vi "Load Program Definition as Table.vi"() -> ()   [LabVIEW 2010]
doc: "This function is an offline tool for importing MICS Command and Response Tables from Excel. \n\nInstructions\n1) Copy clipboard from Excel to Import Control.\n2) Run VI.\n3) Edit - Make Current Values Defaults.\n4) Save VI.\n5) Copy tables to new VIs."
panel:
  out "error out":errorcluster
  in  "error in":errorcluster
  in  "Table 2":string[][](table)=[["255", "0xFF", "COMMAND ACCEPTED", "The received command (identified in the response) was processed and performed without error. Any data to be returned as a result of the command completion is present in the response."], ["0", "0x00", "INVALID EXID", "The External ID contained in the command is for an external device the xPG has not been configured to process commands from."], ["1", "0x01", "INVALID COMMAND", "The Token in the received command is invalid/unknown to the xPG."], ["2", "0x02", "INVALID PARAM", "A parameter provided with the received command has been determined to be invalid and prohibits further processing of the command."], ["3", "0x03", "BUSY", "The xPG cannot execute the received command while in its present operational state.  Examples include: * Selecting program while stim on * Restoring program defaults while stim on * Writing to flash while stim on [CP commands] "], ["16", "0x10", "COMMAND NOT VALID WHILE IDLE", "The command is not valid when stimulation is not active.  (This code generally applies to commands that are used to modify stimulation.)"], ["17", "0x11", "COMMAND NOT VALID WHILE RAMPING", "The command is not valid when the xPG is ramping the stimulus amplitude immediately after turning stimulation on.  (This code generally applies to commands that are used to modify stimulation parameters)"], ["18", "0x12", "COMMAND LOCKED OUT (temporary)", "The command is temporarily locked out. (This code generally applies to commands that are used to modify stimulation, resulting in an increase in stimulation energy)"], ["19", "0x13", "DEPRECATED", ""], ["32", "0x20", "PROGRAM NOT VALID", "The command cannot be executed because the program definition is not valid.  A way to delete a program is to set it not valid.  Then when IPG returns valid programs bitmap it will not be listed as available."], ["33", "0x21", "PROGRAM DISABLED", "The command cannot be executed because the program definition has been disabled, due to a hardware issue."], ["34", "0x22", "BATTERY TOO LOW", "The xPG Stimulation command to turn stimulation on cannot be executed because the battery level is too low for safe stimulation.  IPG could have said battery was OK, but then dropped below threshold since having last sent status.  "], ["35", "0x23", "DEPRECATED –  Use 0x03 BUSY. ", ""], ["36", "0x24", "NO PROGRAM SELECTED", "The requested command (only in response to stim on) cannot be executed because no program is presently selected."], ["37", "0x25", "BOOST CONVERTER STARTUP FAILED", "Stimulation cannot be started because the high voltage boost converter did not initialize correctly."], ["38", "0x26", "PULSE GUARD CHECK FAILED", "Stimulation cannot be started because the pulse guard circuit check failed."], ["39", "0x27", "STIMULATION POWER ON FAILED", "Stimulation cannot be started because the stimulation chip failed to power up correctly."], ["40", "0x28", "ACTIVE RECOVERY DISABLED", "Stimulation cannot be started because automatic waveform adjustment failed."], ["41", "0x29", "DEPRECATED – Use 0x36 MOD VIOLATES ELECTRODE CHARGE DENSITY LIMIT", ""], ["42", "0x2A", "DEPRECATED – Use 0x02 INVALID PARAM.", ""], ["43", "0x2B", "DEPRECATED – USE 0x02 INVALID PARAM.", ""], ["44", "0x2C", "DEPRECATED – Use 0x02 INVALID PARAM.", ""], ["45", "0x2D", "DEPRECATED – Use 0x02 INVALID PARAM.", ""], ["46", "0x2E", "SETUP ERROR, BAD STIM ASIC READ-BACK", "While attempting to set-up the stim ASIC for output, the verification data read-back of certain registers did not match the set-up data. "], ["47", "0x2F", "SETUP ERROR, BAD POWER ASIC READ-BACK", "While attempting to configure the power ASIC, the verification data read-back of certain registers did not match the set-up data."], ["48", "0x30", "DEPRECATED – Not Used.", ""], ["49", "0x31", "ALL AMPLITUDES AT MINIMUM", "The Decrement Program Amplitude command cannot be executed because all pulse amplitudes are the minimum allowed setting."], ["50", "0x32", "ALL AMPLITUDES AT MAXIMUM", "The Increment Program Amplitude command cannot be executed because all pulse amplitudes are the maximum allowed setting."], ["51", "0x33", "PULSE NOT VALID", "The command to modify the specified pulse amplitude or pulse width cannot be executed because the pulse in not defined in the program that is running."], ["52", "0x34", "PULSE WIDTH EXCEEDS LIMITS", "The requested pulse width modification command cannot be executed because it would exceed the programmed pulse width limits for the specified pulse."], ["53", "0x35", "DEPRECATED - Use 0x02 INVALID PARAM.", ""], ["54", "0x36", "MOD VIOLATES ELECTRODE CHARGE DENSITY LIMIT", "The requested pulse output modification cannot be executed because it would violate the charge density limit for one or more of the selected electrode channels."], ["55", "0x37", "MOD VIOLATES ELECTRODE CURRENT DENSITY LIMIT", "The requested pulse output modification cannot be executed because it would violate the current density limit for one or more of the selected electrode channels."], ["56", "0x38", "PULSE WIDTH FREQUENCY CONFLICT", "* The requested pulse width increase cannot be executed because the program cannot be implemented at the specified program frequency. * The requested program frequency increase cannot be executed because the program cannot be implemented with the specified pulse widths. * The requested Test Pulse will not fit in the selected program period. * The requested pulse output requires active recovery, but the KrecsEnabledBitMap in the Pulse Constants is 0 (no krecs enabled). * The requested pulse output requires active recovery, but there are no krecs enabled (KrecsEnabledBitMap in Pulse Constants) that will fit the selected program period. "], ["57", "0x39", "DEPRECATED – Use PULSE WIDTH FREQUENCY CONFLICT", ""], ["58", "0x3A", "FREQUENCY MOD NOT ALLOWED", "The requested program frequency change is not allowed per the program definition.  (This could be because the specified frequency is not allowed or there is no frequency index lower or higher than the present index allowed.)"], ["59", "0x3B", "PULSE AMPLITUDE EXCEEDS LIMITS", "The requested pulse amplitude change cannot be executed because it would exceed the allowed limits for the specified pulse."], ["60", "0x3C", "DEPRECATED – Command n long exists", ""], ["64", "0x40", "TIMED OUT", "The operation requested timed out waiting for hardware to respond.  This response includes when an ADC read fails or when background impedance check fails to respond with a value."], ["85", "0x55", "CHARGING CONTROL ERROR", "An error occurred reading the temperature or battery level."], ["96", "0x60", "DATA CORRUPTED", "The requested Get Data command failed, or the requested data was detected as corrupt."], ["97", "0x61", "PROGRAM DEFINITION CORRUPTED", "The data integrity check for the program definition data for the requested program failed. IPG should set active error to PROGRAM DEFINITION CORRUPTED"], ["98", "0x62", "PROGRAM ACTIVE SETTINGS CORRUPTED", "The data integrity check for the active settings for the requested program failed.  IPG should set active error to PROGRAM ACTIVE SETTINGS CORRUPTED.  IPG will also return that active settings to default settings."], ["99", "0x63", "PROGRAM CONSTANTS CORRUPTED", "The data integrity check for the Program Constants data failed.  xPG should set active error to CRITICAL NV DATA CORRUPTED."], ["100", "0x64", "PULSE CONSTANTS CORRUPTED", "The data integrity check for the Pulse Constants data failed.  xPG should set active error to CRITICAL NV DATA CORRUPTED."], ["101", "0x65", "CHANNEL CALIBRATIONS CORRUPTED", "The data integrity check for the Channel Calibrations data failed.  xPG should set active error to CRITICAL NV DATA CORRUPTED."], ["102", "0x66", "LEAD LIMITS CORRUPTED", "The data integrity check for the Lead Limits data failed.  xPG should set active error to CRITICAL NV DATA CORRUPTED."], ["103", "0x67", "STIM ASIC HV CALIBRATIONS CORRUPTED", "The data integrity check for the Stim Asic HV Calibrations data failed.  xPG should set active error to CRITICAL NV DATA CORRUPTED."], ["104", "0x68", "RAMP TIME CORRUPTED", "The data integrity check for the Ramp Time failed.  xPG should set active error to CRITICAL NV DATA CORRUPTED."], ["105", "0x69", "DEPRECATED", ""], ["106", "0x6A", "DEPRECATED – Not Used", ""], ["112", "0x70", "FEATURE NOT ENABLED", "The requested feature is not presently enabled."], ["113", "0x71", "DEPRECATED - Use 0x02 INVALID PARAM.", ""], ["114", "0x72", "DEPRECATED - Use 0x02 INVALID PARAM.", ""], ["115", "0x73", "DEPRECATED – Use 0x03 BUSY.", ""], ["116", "0x74", "DEPRECATED – Use 0x38 PULSE WIDTH FREQUENCY CONFLICT", ""], ["117", "0x75", "DEPRECATED – Use 0x38 PULSE WIDTH FREQUENCY CONFLICT", ""], ["118", "0x76", "DEPRECATED – Use 0x38 PULSE WIDTH FREQUENCY CONFLICT", ""], ["119", "0x77", "WRITE FAILED", "The command failed while attempting to write data to memory or registers. Writes to flash shall use more specific error codes from the range below."], ["120", "0x78", "READ FAILED", "The command failed while attempting to read data to memory or registers. Reads to flash shall use more specific error codes from the range below."], ["121", "0x79", "DEPRECATED – Not Used", ""], ["128", "0x80", "DEPRECATED – Not Used", ""], ["129", "0x81", "BACKGROUND IMPEDANCE CHECK FAILED", "Pre-stimulation background impedance checks have failed.  This shall result in a Category 2 Error being reported."], ["130", "0x82", "BASIC OUTPUT CHECK FAILED", "Pre-stimulation basic output checks have failed.  This shall result in a Category 2 Error being reported."], ["131", "0x83", "STIM FAILED UNKNOWN SOFTWARE ERROR", "Stimulation has failed because of a software logic error.  Stimulation cannot be started."], ["132", "0x84", "STIMULATION FAILED – SEVERE ERROR EXISTS", "Stimulation has failed because a Category 1 error exists.  Stimulation cannot be started if such an error exists."], ["133", "0x85", "DEPRECATED – Not Used", ""], ["176", "0xB0", "FLASH ERROR INVALID ADDRESS", "Illegal flash address segment write.  The requested programming command failed while attempting to save data to the xPG’s non-volatile memory."], ["177", "0xB1", "FLASH ERROR SEGMENT BOUNDARY", "Requested flash address write overlaps segment boundary.  The requested programming command failed while attempting to save data to the xPG’s non-volatile memory."], ["178", "0xB2", "DEPRECATED – Use 0xB0 FLASH ERROR INVALID ADDRESS", "Invalid flash address reported while preparing for erasing segment.  The requested programming command failed while attempting to save data to the xPG’s non-volatile memory."], ["179", "0xB3", "FLASH ERASE ERROR FLASH CONTROLLER BUSY", "Flash controller unexpectedly reported busy while preparing for segment erase.  The requested programming command failed while attempting to save data to the xPG’s non-volatile memory."], ["180", "0xB4", "FLASH ERASE ERROR FLASH CONTROLLER SETUP", "Firmware setup error reported while preparing for segment erase.  The requested programming command failed while attempting to save data to the xPG’s non-volatile memory."], ["181", "0xB5", "FLASH ERASE ERROR TIMEOUT", "Busy bit timeout reported while waiting for segment erase. The requested programming command failed while attempting to save data to the xPG’s non-volatile memory."], ["182", "0xB6", "FLASH ERASE ERROR FAIL FLAG", "Fail flag set during segment erase.  The requested programming command failed while attempting to save data to the xPG’s non-volatile memory."], ["183", "0xB7", "FLASH ERASE ERROR ACCESS VIOLATION FLAG", "Access violation reported while attempting to erase flash.  The requested programming command failed while attempting to save data to the xPG’s non-volatile memory."], ["184", "0xB8", "FLASH ERASE ERROR BAD ERASE", "Segment not erased and segment erase reported as completed.  The requested programming command failed while attempting to save data to the xPG’s non-volatile memory."], ["192", "0xC0", "DEPRECATED – Use 0xB0 FLASH ERROR INVALID ADDRESS", ""], ["193", "0xC1", "FLASH WRITE ERROR FLASH CONTROLLER BUSY", "The flash controller reports unexpectedly busy while preparing for block write.  The requested programming command failed while attempting to save data to the xPG’s non-volatile memory."], ["194", "0xC2", "FLASH WRITE ERROR FLASH CONTROLLER SETUP", "A firmware setup error occurred while preparing for block write.  The requested programming command failed while attempting to save data to the xPG’s non-volatile memory."], ["195", "0xC3", "FLASH WORD WRITE ERROR TIMEOUT", "Wait bit timeout occurred while writing word to flash memory.  The requested programming command failed while attempting to save data to the xPG’s non-volatile memory."], ["196", "0xC4", "FLASH  WORD WRITE ERROR FAIL FLAG", "Flash fail flag set while writing word to flash memory.  The requested programming command failed while attempting to save data to the xPG’s non-volatile memory."], ["197", "0xC5", "FLASH WORD WRITE ERROR ACCESS VIOLATION", "Access violation reported while writing word to flash memory.  The requested programming command failed while attempting to save data to the xPG’s non-volatile memory."], ["198", "0xC6", "FLASH BLOCK WRITE ERROR TIMEOUT", "Wait bit timeout occurred while writing block to flash memory.  The requested programming command failed while attempting to save data to the xPG’s non-volatile memory."], ["199", "0xC7", "FLASH  BLOCK WRITE ERROR FAIL FLAG", "Flash fail flag set while writing block to flash memory.  The requested programming command failed while attempting to save data to the xPG’s non-volatile memory."], ["200", "0xC8", "FLASH BLOCK WRITE ERROR ACCESS VIOLATION", "Access violation reported while writing block to flash memory.  The requested programming command failed while attempting to save data to the xPG’s non-volatile memory."], ["201", "0xC9", "FLASH WRITE ERROR BAD WRITE", "After segment write completed, the flash destination data did not match the source data.  The requested programming command failed while attempting to save data to the xPG’s non-volatile memory."], ["202", "0xCA", "RESERVED – Not Used.", ""], ["203", "0xCB", "RESERVED – Not Used.", ""], ["204", "0xCC", "RESERVED – Not Used.", ""], ["205", "0xCD", "RESERVED – Not Used.", ""], ["206", "0xCE", "RESERVED – Not Used.", ""], ["207", "0xCF", "RESERVED – Not Used.", ""], ["-1", "Default", "ANY ERROR NOT LISTED HEREIN", "Undefined and unexpected.   "]]
  in  "Excel Clipboard to Import 2":string="255\t0xFF\tCOMMAND ACCEPTED\tThe received command (identified in the response) was processed and performed without error. Any data to be returned as a result of the command completion is present in the response.\n0\t0x00\tINVALID EXID\tThe External ID contained in the command is for an external device the xPG has not been configured to process commands from.\n1\t0x01\tINVALID COMMAND\tThe Token in the received command is invalid/unknown to the xPG.\n2\t0x02\tINVALID PARAM\tA parameter provided with the received command has been determined to be invalid and prohibits further processing of the command.\n3\t0x03\tBUSY\tThe xPG cannot execute the received command while in its present operational state.  Examples include: * Selecting program while stim on * Restoring program defaults while stim on * Writing to flash while stim on [CP commands] \n16\t0x10\tCOMMAND NOT VALID WHILE IDLE\tThe command is not valid when stimulation is not active.  (This code generally applies to commands that are used to modify stimulation.)\n17\t0x11\tCOMMAND NOT VALID WHILE RAMPING\tThe command is not valid when the xPG is ramping the stimulus amplitude immediately after turning stimulation on.  (This code generally applies to commands that are used to modify stimulation parameters)\n18\t0x12\tCOMMAND LOCKED OUT (temporary)\tThe command is temporarily locked out. (This code generally applies to commands that are used to modify stimulation, resulting in an increase in stimulation energy)\n19\t0x13\tDEPRECATED\t\n32\t0x20\tPROGRAM NOT VALID\tThe command cannot be executed because the program definition is not valid.  A way to delete a program is to set it not valid.  Then when IPG returns valid programs bitmap it will not be listed as available.\n33\t0x21\tPROGRAM DISABLED\tThe command cannot be executed because the program definition has been disabled, due to a hardware issue.\n34\t0x22\tBATTERY TOO LOW\tThe xPG Stimulation command to turn stimulation on cannot be executed because the battery level is too low for safe stimulation.  IPG could have said battery was OK, but then dropped below threshold since having last sent status.  \n35\t0x23\tDEPRECATED –  Use 0x03 BUSY. \t\n36\t0x24\tNO PROGRAM SELECTED\tThe requested command (only in response to stim on) cannot be executed because no program is presently selected.\n37\t0x25\tBOOST CONVERTER STARTUP FAILED\tStimulation cannot be started because the high voltage boost converter did not initialize correctly.\n38\t0x26\tPULSE GUARD CHECK FAILED\tStimulation cannot be started because the pulse guard circuit check failed.\n39\t0x27\tSTIMULATION POWER ON FAILED\tStimulation cannot be started because the stimulation chip failed to power up correctly.\n40\t0x28\tACTIVE RECOVERY DISABLED\tStimulation cannot be started because automatic waveform adjustment failed.\n41\t0x29\tDEPRECATED – Use 0x36 MOD VIOLATES ELECTRODE CHARGE DENSITY LIMIT\t\n42\t0x2A\tDEPRECATED – Use 0x02 INVALID PARAM.\t\n43\t0x2B\tDEPRECATED – USE 0x02 INVALID PARAM.\t\n44\t0x2C\tDEPRECATED – Use 0x02 INVALID PARAM.\t\n45\t0x2D\tDEPRECATED – Use 0x02 INVALID PARAM.\t\n46\t0x2E\tSETUP ERROR, BAD STIM ASIC READ-BACK\tWhile attempting to set-up the stim ASIC for output, the verification data read-back of certain registers did not match the set-up data. \n47\t0x2F\tSETUP ERROR, BAD POWER ASIC READ-BACK\tWhile attempting to configure the power ASIC, the verification data read-back of certain registers did not match the set-up data.\n48\t0x30\tDEPRECATED – Not Used.\t\n49\t0x31\tALL AMPLITUDES AT MINIMUM\tThe Decrement Program Amplitude command cannot be executed because all pulse amplitudes are the minimum allowed setting.\n50\t0x32\tALL AMPLITUDES AT MAXIMUM\tThe Increment Program Amplitude command cannot be executed because all pulse amplitudes are the maximum allowed setting.\n51\t0x33\tPULSE NOT VALID\tThe command to modify the specified pulse amplitude or pulse width cannot be executed because the pulse in not defined in the program that is running.\n52\t0x34\tPULSE WIDTH EXCEEDS LIMITS\tThe requested pulse width modification command cannot be executed because it would exceed the programmed pulse width limits for the specified pulse.\n53\t0x35\tDEPRECATED - Use 0x02 INVALID PARAM.\t\n54\t0x36\tMOD VIOLATES ELECTRODE CHARGE DENSITY LIMIT\tThe requested pulse output modification cannot be executed because it would violate the charge density limit for one or more of the selected electrode channels.\n55\t0x37\tMOD VIOLATES ELECTRODE CURRENT DENSITY LIMIT\tThe requested pulse output modification cannot be executed because it would violate the current density limit for one or more of the selected electrode channels.\n56\t0x38\tPULSE WIDTH FREQUENCY CONFLICT\t* The requested pulse width increase cannot be executed because the program cannot be implemented at the specified program frequency. * The requested program frequency increase cannot be executed because the program cannot be implemented with the specified pulse widths. * The requested Test Pulse will not fit in the selected program period. * The requested pulse output requires active recovery, but the KrecsEnabledBitMap in the Pulse Constants is 0 (no krecs enabled). * The requested pulse output requires active recovery, but there are no krecs enabled (KrecsEnabledBitMap in Pulse Constants) that will fit the selected program period. \n57\t0x39\tDEPRECATED – Use PULSE WIDTH FREQUENCY CONFLICT\t\n58\t0x3A\tFREQUENCY MOD NOT ALLOWED\tThe requested program frequency change is not allowed per the program definition.  (This could be because the specified frequency is not allowed or there is no frequency index lower or higher than the present index allowed.)\n59\t0x3B\tPULSE AMPLITUDE EXCEEDS LIMITS\tThe requested pulse amplitude change cannot be executed because it would exceed the allowed limits for the specified pulse.\n60\t0x3C\tDEPRECATED – Command n long exists\t\n64\t0x40\tTIMED OUT\tThe operation requested timed out waiting for hardware to respond.  This response includes when an ADC read fails or when background impedance check fails to respond with a value.\n85\t0x55\tCHARGING CONTROL ERROR\tAn error occurred reading the temperature or battery level.\n96\t0x60\tDATA CORRUPTED\tThe requested Get Data command failed, or the requested data was detected as corrupt.\n97\t0x61\tPROGRAM DEFINITION CORRUPTED\tThe data integrity check for the program definition data for the requested program failed. IPG should set active error to PROGRAM DEFINITION CORRUPTED\n98\t0x62\tPROGRAM ACTIVE SETTINGS CORRUPTED\tThe data integrity check for the active settings for the requested program failed.  IPG should set active error to PROGRAM ACTIVE SETTINGS CORRUPTED.  IPG will also return that active settings to default settings.\n99\t0x63\tPROGRAM CONSTANTS CORRUPTED\tThe data integrity check for the Program Constants data failed.  xPG should set active error to CRITICAL NV DATA CORRUPTED.\n100\t0x64\tPULSE CONSTANTS CORRUPTED\tThe data integrity check for the Pulse Constants data failed.  xPG should set active error to CRITICAL NV DATA CORRUPTED.\n101\t0x65\tCHANNEL CALIBRATIONS CORRUPTED\tThe data integrity check for the Channel Calibrations data failed.  xPG should set active error to CRITICAL NV DATA CORRUPTED.\n102\t0x66\tLEAD LIMITS CORRUPTED\tThe data integrity check for the Lead Limits data failed.  xPG should set active error to CRITICAL NV DATA CORRUPTED.\n103\t0x67\tSTIM ASIC HV CALIBRATIONS CORRUPTED\tThe data integrity check for the Stim Asic HV Calibrations data failed.  xPG should set active error to CRITICAL NV DATA CORRUPTED.\n104\t0x68\tRAMP TIME CORRUPTED\tThe data integrity check for the Ramp Time failed.  xPG should set active error to CRITICAL NV DATA CORRUPTED.\n105\t0x69\tDEPRECATED\t\n106\t0x6A\tDEPRECATED – Not Used\t\n112\t0x70\tFEATURE NOT ENABLED\tThe requested feature is not presently enabled.\n113\t0x71\tDEPRECATED - Use 0x02 INVALID PARAM.\t\n114\t0x72\tDEPRECATED - Use 0x02 INVALID PARAM.\t\n115\t0x73\tDEPRECATED – Use 0x03 BUSY.\t\n116\t0x74\tDEPRECATED – Use 0x38 PULSE WIDTH FREQUENCY CONFLICT\t\n117\t0x75\tDEPRECATED – Use 0x38 PULSE WIDTH FREQUENCY CONFLICT\t\n118\t0x76\tDEPRECATED – Use 0x38 PULSE WIDTH FREQUENCY CONFLICT\t\n119\t0x77\tWRITE FAILED\tThe command failed while attempting to write data to memory or registers. Writes to flash shall use more specific error codes from the range below.\n120\t0x78\tREAD FAILED\tThe command failed while attempting to read data to memory or registers. Reads to flash shall use more specific error codes from the range below.\n121\t0x79\tDEPRECATED – Not Used\t\n128\t0x80\tDEPRECATED – Not Used\t\n129\t0x81\tBACKGROUND IMPEDANCE CHECK FAILED\tPre-stimulation background impedance checks have failed.  This shall result in a Category 2 Error being reported.\n130\t0x82\tBASIC OUTPUT CHECK FAILED\tPre-stimulation basic output checks have failed.  This shall result in a Category 2 Error being reported.\n131\t0x83\tSTIM FAILED UNKNOWN SOFTWARE ERROR\tStimulation has failed because of a software logic error.  Stimulation cannot be started.\n132\t0x84\tSTIMULATION FAILED – SEVERE ERROR EXISTS\tStimulation has failed because a Category 1 error exists.  Stimulation cannot be started if such an error exists.\n133\t0x85\tDEPRECATED – Not Used\t\n176\t0xB0\tFLASH ERROR INVALID ADDRESS\tIllegal flash address segment write.  The requested programming command failed while attempting to save data to the xPG’s non-volatile memory.\n177\t0xB1\tFLASH ERROR SEGMENT BOUNDARY\tRequested flash address write overlaps segment boundary.  The requested programming command failed while attempting to save data to the xPG’s non-volatile memory.\n178\t0xB2\tDEPRECATED – Use 0xB0 FLASH ERROR INVALID ADDRESS\tInvalid flash address reported while preparing for erasing segment.  The requested programming command failed while attempting to save data to the xPG’s non-volatile memory.\n179\t0xB3\tFLASH ERASE ERROR FLASH CONTROLLER BUSY\tFlash controller unexpectedly reported busy while preparing for segment erase.  The requested programming command failed while attempting to save data to the xPG’s non-volatile memory.\n180\t0xB4\tFLASH ERASE ERROR FLASH CONTROLLER SETUP\tFirmware setup error reported while preparing for segment erase.  The requested programming command failed while attempting to save data to the xPG’s non-volatile memory.\n181\t0xB5\tFLASH ERASE ERROR TIMEOUT\tBusy bit timeout reported while waiting for segment erase. The requested programming command failed while attempting to save data to the xPG’s non-volatile memory.\n182\t0xB6\tFLASH ERASE ERROR FAIL FLAG\tFail flag set during segment erase.  The requested programming command failed while attempting to save data to the xPG’s non-volatile memory.\n183\t0xB7\tFLASH ERASE ERROR ACCESS VIOLATION FLAG\tAccess violation reported while attempting to erase flash.  The requested programming command failed while attempting to save data to the xPG’s non-volatile memory.\n184\t0xB8\tFLASH ERASE ERROR BAD ERASE\tSegment not erased and segment erase reported as completed.  The requested programming command failed while attempting to save data to the xPG’s non-volatile memory.\n192\t0xC0\tDEPRECATED – Use 0xB0 FLASH ERROR INVALID ADDRESS\t\n193\t0xC1\tFLASH WRITE ERROR FLASH CONTROLLER BUSY\tThe flash controller reports unexpectedly busy while preparing for block write.  The requested programming command failed while attempting to save data to the xPG’s non-volatile memory.\n194\t0xC2\tFLASH WRITE ERROR FLASH CONTROLLER SETUP\tA firmware setup error occurred while preparing for block write.  The requested programming command failed while attempting to save data to the xPG’s non-volatile memory.\n195\t0xC3\tFLASH WORD WRITE ERROR TIMEOUT\tWait bit timeout occurred while writing word to flash memory.  The requested programming command failed while attempting to save data to the xPG’s non-volatile memory.\n196\t0xC4\tFLASH  WORD WRITE ERROR FAIL FLAG\tFlash fail flag set while writing word to flash memory.  The requested programming command failed while attempting to save data to the xPG’s non-volatile memory.\n197\t0xC5\tFLASH WORD WRITE ERROR ACCESS VIOLATION\tAccess violation reported while writing word to flash memory.  The requested programming command failed while attempting to save data to the xPG’s non-volatile memory.\n198\t0xC6\tFLASH BLOCK WRITE ERROR TIMEOUT\tWait bit timeout occurred while writing block to flash memory.  The requested programming command failed while attempting to save data to the xPG’s non-volatile memory.\n199\t0xC7\tFLASH  BLOCK WRITE ERROR FAIL FLAG\tFlash fail flag set while writing block to flash memory.  The requested programming command failed while attempting to save data to the xPG’s non-volatile memory.\n200\t0xC8\tFLASH BLOCK WRITE ERROR ACCESS VIOLATION\tAccess violation reported while writing block to flash memory.  The requested programming command failed while attempting to save data to the xPG’s non-volatile memory.\n201\t0xC9\tFLASH WRITE ERROR BAD WRITE\tAfter segment write completed, the flash destination data did not match the source data.  The requested programming command failed while attempting to save data to the xPG’s non-volatile memory.\n202\t0xCA\tRESERVED – Not Used.\t\n203\t0xCB\tRESERVED – Not Used.\t\n204\t0xCC\tRESERVED – Not Used.\t\n205\t0xCD\tRESERVED – Not Used.\t\n206\t0xCE\tRESERVED – Not Used.\t\n207\t0xCF\tRESERVED – Not Used.\t\n-1\tDefault\tANY ERROR NOT LISTED HEREIN\tUndefined and unexpected.   \n"
  in  "Excel Clipboard1 to Import 1":string="ProgramNumber\t2\nProgramDefined\t1\nProgramDisabled\t0\nProgramName\tP-A Switching02\nAllowedFrequencies[0]\t0x00\nAllowedFrequencies[1]\t0x00\nAllowedFrequencies[2]\t0x00\nAllowedFrequencies[3]\t0xFF\nAllowedFrequencies[4]\t0x00\nAllowedFrequencies[5]\t0x00\nAllowedFrequencies[6]\t0x00\nAllowedFrequencies[7]\t0x00\nProgramFrequencyIndex\t29\nDefinedPulseMap\t3\nPulseNamePA\tP1\nAmplitudeLowLimitPA\t5000\nAmplitudeStepPA\t15\nAmplitudeStepIndexPA\t1\nPulseWidthLowLimitPA\t900\nPulseWidthHighLimitPA\t1000\nPulseWidthPA\t950\nElectrodeAmpPercentagePA[CH01]\t0\nElectrodeAmpPercentagePA[CH02]\t0\nElectrodeAmpPercentagePA[CH03]\t0\nElectrodeAmpPercentagePA[CH04]\t0\nElectrodeAmpPercentagePA[CH05]\t0\nElectrodeAmpPercentagePA[CH06]\t0\nElectrodeAmpPercentagePA[CH07]\t0\nElectrodeAmpPercentagePA[CH08]\t0\nElectrodeAmpPercentagePA[CH09]\t0\nElectrodeAmpPercentagePA[CH10]\t0\nElectrodeAmpPercentagePA[CH11]\t0\nElectrodeAmpPercentagePA[CH12]\t0\nElectrodeAmpPercentagePA[CH13]\t0\nElectrodeAmpPercentagePA[CH14]\t0\nElectrodeAmpPercentagePA[CH15]\t0\nElectrodeAmpPercentagePA[CH16]\t100\nElectrodeAmpPercentagePA[CH17]\t-100\nElectrodeAmpPercentagePA[CH18]\t0\nElectrodeAmpPercentagePA[CH19]\t0\nElectrodeAmpPercentagePA[CH20]\t0\nElectrodeAmpPercentagePA[CH21]\t0\nElectrodeAmpPercentagePA[CH22]\t0\nElectrodeAmpPercentagePA[CH23]\t0\nElectrodeAmpPercentagePA[CH24]\t0\nElectrodeAmpPercentagePA[CH25]\t0\nElectrodeAmpPercentagePA[CH26]\t0\nPulseNamePB\tP2\nAmplitudeLowLimitPB\t4000\nAmplitudeStepPB\t15\nAmplitudeStepIndexPB\t1\nPulseWidthLowLimitPB\t900\nPulseWidthHighLimitPB\t1100\nPulseWidthPB\t1000\nElectrodeAmpPercentagePB[CH01]\t0\nElectrodeAmpPercentagePB[CH02]\t0\nElectrodeAmpPercentagePB[CH03]\t0\nElectrodeAmpPercentagePB[CH04]\t0\nElectrodeAmpPercentagePB[CH05]\t0\nElectrodeAmpPercentagePB[CH06]\t0\nElectrodeAmpPercentagePB[CH07]\t0\nElectrodeAmpPercentagePB[CH08]\t0\nElectrodeAmpPercentagePB[CH09]\t0\nElectrodeAmpPercentagePB[CH10]\t0\nElectrodeAmpPercentagePB[CH11]\t0\nElectrodeAmpPercentagePB[CH12]\t0\nElectrodeAmpPercentagePB[CH13]\t0\nElectrodeAmpPercentagePB[CH14]\t0\nElectrodeAmpPercentagePB[CH15]\t0\nElectrodeAmpPercentagePB[CH16]\t100\nElectrodeAmpPercentagePB[CH17]\t-100\nElectrodeAmpPercentagePB[CH18]\t0\nElectrodeAmpPercentagePB[CH19]\t0\nElectrodeAmpPercentagePB[CH20]\t0\nElectrodeAmpPercentagePB[CH21]\t0\nElectrodeAmpPercentagePB[CH22]\t0\nElectrodeAmpPercentagePB[CH23]\t0\nElectrodeAmpPercentagePB[CH24]\t0\nElectrodeAmpPercentagePB[CH25]\t0\nElectrodeAmpPercentagePB[CH26]\t0\nPulseNamePC\t0\nAmplitudeLowLimitPC\t0\nAmplitudeStepPC\t15\nAmplitudeStepIndexPC\t0\nPulseWidthLowLimitPC\t0\nPulseWidthHighLimitPC\t0\nPulseWidthPC\t0\nElectrodeAmpPercentagePC[CH01]\t0\nElectrodeAmpPercentagePC[CH02]\t0\nElectrodeAmpPercentagePC[CH03]\t0\nElectrodeAmpPercentagePC[CH04]\t0\nElectrodeAmpPercentagePC[CH05]\t0\nElectrodeAmpPercentagePC[CH06]\t0\nElectrodeAmpPercentagePC[CH07]\t0\nElectrodeAmpPercentagePC[CH08]\t0\nElectrodeAmpPercentagePC[CH09]\t0\nElectrodeAmpPercentagePC[CH10]\t0\nElectrodeAmpPercentagePC[CH11]\t0\nElectrodeAmpPercentagePC[CH12]\t0\nElectrodeAmpPercentagePC[CH13]\t0\nElectrodeAmpPercentagePC[CH14]\t0\nElectrodeAmpPercentagePC[CH15]\t0\nElectrodeAmpPercentagePC[CH16]\t0\nElectrodeAmpPercentagePC[CH17]\t0\nElectrodeAmpPercentagePC[CH18]\t0\nElectrodeAmpPercentagePC[CH19]\t0\nElectrodeAmpPercentagePC[CH20]\t0\nElectrodeAmpPercentagePC[CH21]\t0\nElectrodeAmpPercentagePC[CH22]\t0\nElectrodeAmpPercentagePC[CH23]\t0\nElectrodeAmpPercentagePC[CH24]\t0\nElectrodeAmpPercentagePC[CH25]\t0\nElectrodeAmpPercentagePC[CH26]\t0\nPulseNamePD\t0\nAmplitudeLowLimitPD\t0\nAmplitudeStepPD\t15\nAmplitudeStepIndexPD\t0\nPulseWidthLowLimitPD\t0\nPulseWidthHighLimitPD\t0\nPulseWidthPD\t0\nElectrodeAmpPercentagePD[CH01]\t0\nElectrodeAmpPercentagePD[CH02]\t0\nElectrodeAmpPercentagePD[CH03]\t0\nElectrodeAmpPercentagePD[CH04]\t0\nElectrodeAmpPercentagePD[CH05]\t0\nElectrodeAmpPercentagePD[CH06]\t0\nElectrodeAmpPercentagePD[CH07]\t0\nElectrodeAmpPercentagePD[CH08]\t0\nElectrodeAmpPercentagePD[CH09]\t0\nElectrodeAmpPercentagePD[CH10]\t0\nElectrodeAmpPercentagePD[CH11]\t0\nElectrodeAmpPercentagePD[CH12]\t0\nElectrodeAmpPercentagePD[CH13]\t0\nElectrodeAmpPercentagePD[CH14]\t0\nElectrodeAmpPercentagePD[CH15]\t0\nElectrodeAmpPercentagePD[CH16]\t0\nElectrodeAmpPercentagePD[CH17]\t0\nElectrodeAmpPercentagePD[CH18]\t0\nElectrodeAmpPercentagePD[CH19]\t0\nElectrodeAmpPercentagePD[CH20]\t0\nElectrodeAmpPercentagePD[CH21]\t0\nElectrodeAmpPercentagePD[CH22]\t0\nElectrodeAmpPercentagePD[CH23]\t0\nElectrodeAmpPercentagePD[CH24]\t0\nElectrodeAmpPercentagePD[CH25]\t0\nElectrodeAmpPercentagePD[CH26]\t0\n"
  in  "Table 1":string[][](table)=[["ProgramNumber", "2"], ["ProgramDefined", "1"], ["ProgramDisabled", "0"], ["ProgramName", "P-A Switching02"], ["AllowedFrequencies[0]", "0x00"], ["AllowedFrequencies[1]", "0x00"], ["AllowedFrequencies[2]", "0x00"], ["AllowedFrequencies[3]", "0xFF"], ["AllowedFrequencies[4]", "0x00"], ["AllowedFrequencies[5]", "0x00"], ["AllowedFrequencies[6]", "0x00"], ["AllowedFrequencies[7]", "0x00"], ["ProgramFrequencyIndex", "29"], ["DefinedPulseMap", "3"], ["PulseNamePA", "P1"], ["AmplitudeLowLimitPA", "5000"], ["AmplitudeStepPA", "15"], ["AmplitudeStepIndexPA", "1"], ["PulseWidthLowLimitPA", "900"], ["PulseWidthHighLimitPA", "1000"], ["PulseWidthPA", "950"], ["ElectrodeAmpPercentagePA[CH01]", "0"], ["ElectrodeAmpPercentagePA[CH02]", "0"], ["ElectrodeAmpPercentagePA[CH03]", "0"], ["ElectrodeAmpPercentagePA[CH04]", "0"], ["ElectrodeAmpPercentagePA[CH05]", "0"], ["ElectrodeAmpPercentagePA[CH06]", "0"], ["ElectrodeAmpPercentagePA[CH07]", "0"], ["ElectrodeAmpPercentagePA[CH08]", "0"], ["ElectrodeAmpPercentagePA[CH09]", "0"], ["ElectrodeAmpPercentagePA[CH10]", "0"], ["ElectrodeAmpPercentagePA[CH11]", "0"], ["ElectrodeAmpPercentagePA[CH12]", "0"], ["ElectrodeAmpPercentagePA[CH13]", "0"], ["ElectrodeAmpPercentagePA[CH14]", "0"], ["ElectrodeAmpPercentagePA[CH15]", "0"], ["ElectrodeAmpPercentagePA[CH16]", "100"], ["ElectrodeAmpPercentagePA[CH17]", "-100"], ["ElectrodeAmpPercentagePA[CH18]", "0"], ["ElectrodeAmpPercentagePA[CH19]", "0"], ["ElectrodeAmpPercentagePA[CH20]", "0"], ["ElectrodeAmpPercentagePA[CH21]", "0"], ["ElectrodeAmpPercentagePA[CH22]", "0"], ["ElectrodeAmpPercentagePA[CH23]", "0"], ["ElectrodeAmpPercentagePA[CH24]", "0"], ["ElectrodeAmpPercentagePA[CH25]", "0"], ["ElectrodeAmpPercentagePA[CH26]", "0"], ["PulseNamePB", "P2"], ["AmplitudeLowLimitPB", "4000"], ["AmplitudeStepPB", "15"], ["AmplitudeStepIndexPB", "1"], ["PulseWidthLowLimitPB", "900"], ["PulseWidthHighLimitPB", "1100"], ["PulseWidthPB", "1000"], ["ElectrodeAmpPercentagePB[CH01]", "0"], ["ElectrodeAmpPercentagePB[CH02]", "0"], ["ElectrodeAmpPercentagePB[CH03]", "0"], ["ElectrodeAmpPercentagePB[CH04]", "0"], ["ElectrodeAmpPercentagePB[CH05]", "0"], ["ElectrodeAmpPercentagePB[CH06]", "0"], ["ElectrodeAmpPercentagePB[CH07]", "0"], ["ElectrodeAmpPercentagePB[CH08]", "0"], ["ElectrodeAmpPercentagePB[CH09]", "0"], ["ElectrodeAmpPercentagePB[CH10]", "0"], ["ElectrodeAmpPercentagePB[CH11]", "0"], ["ElectrodeAmpPercentagePB[CH12]", "0"], ["ElectrodeAmpPercentagePB[CH13]", "0"], ["ElectrodeAmpPercentagePB[CH14]", "0"], ["ElectrodeAmpPercentagePB[CH15]", "0"], ["ElectrodeAmpPercentagePB[CH16]", "100"], ["ElectrodeAmpPercentagePB[CH17]", "-100"], ["ElectrodeAmpPercentagePB[CH18]", "0"], ["ElectrodeAmpPercentagePB[CH19]", "0"], ["ElectrodeAmpPercentagePB[CH20]", "0"], ["ElectrodeAmpPercentagePB[CH21]", "0"], ["ElectrodeAmpPercentagePB[CH22]", "0"], ["ElectrodeAmpPercentagePB[CH23]", "0"], ["ElectrodeAmpPercentagePB[CH24]", "0"], ["ElectrodeAmpPercentagePB[CH25]", "0"], ["ElectrodeAmpPercentagePB[CH26]", "0"], ["PulseNamePC", "0"], ["AmplitudeLowLimitPC", "0"], ["AmplitudeStepPC", "15"], ["AmplitudeStepIndexPC", "0"], ["PulseWidthLowLimitPC", "0"], ["PulseWidthHighLimitPC", "0"], ["PulseWidthPC", "0"], ["ElectrodeAmpPercentagePC[CH01]", "0"], ["ElectrodeAmpPercentagePC[CH02]", "0"], ["ElectrodeAmpPercentagePC[CH03]", "0"], ["ElectrodeAmpPercentagePC[CH04]", "0"], ["ElectrodeAmpPercentagePC[CH05]", "0"], ["ElectrodeAmpPercentagePC[CH06]", "0"], ["ElectrodeAmpPercentagePC[CH07]", "0"], ["ElectrodeAmpPercentagePC[CH08]", "0"], ["ElectrodeAmpPercentagePC[CH09]", "0"], ["ElectrodeAmpPercentagePC[CH10]", "0"], ["ElectrodeAmpPercentagePC[CH11]", "0"], ["ElectrodeAmpPercentagePC[CH12]", "0"], ["ElectrodeAmpPercentagePC[CH13]", "0"], ["ElectrodeAmpPercentagePC[CH14]", "0"], ["ElectrodeAmpPercentagePC[CH15]", "0"], ["ElectrodeAmpPercentagePC[CH16]", "0"], ["ElectrodeAmpPercentagePC[CH17]", "0"], ["ElectrodeAmpPercentagePC[CH18]", "0"], ["ElectrodeAmpPercentagePC[CH19]", "0"], ["ElectrodeAmpPercentagePC[CH20]", "0"], ["ElectrodeAmpPercentagePC[CH21]", "0"], ["ElectrodeAmpPercentagePC[CH22]", "0"], ["ElectrodeAmpPercentagePC[CH23]", "0"], ["ElectrodeAmpPercentagePC[CH24]", "0"], ["ElectrodeAmpPercentagePC[CH25]", "0"], ["ElectrodeAmpPercentagePC[CH26]", "0"], ["PulseNamePD", "0"], ["AmplitudeLowLimitPD", "0"], ["AmplitudeStepPD", "15"], ["AmplitudeStepIndexPD", "0"], ["PulseWidthLowLimitPD", "0"], ["PulseWidthHighLimitPD", "0"], ["PulseWidthPD", "0"], ["ElectrodeAmpPercentagePD[CH01]", "0"], ["ElectrodeAmpPercentagePD[CH02]", "0"], ["ElectrodeAmpPercentagePD[CH03]", "0"], ["ElectrodeAmpPercentagePD[CH04]", "0"], ["ElectrodeAmpPercentagePD[CH05]", "0"], ["ElectrodeAmpPercentagePD[CH06]", "0"], ["ElectrodeAmpPercentagePD[CH07]", "0"], ["ElectrodeAmpPercentagePD[CH08]", "0"], ["ElectrodeAmpPercentagePD[CH09]", "0"], ["ElectrodeAmpPercentagePD[CH10]", "0"], ["ElectrodeAmpPercentagePD[CH11]", "0"], ["ElectrodeAmpPercentagePD[CH12]", "0"], ["ElectrodeAmpPercentagePD[CH13]", "0"], ["ElectrodeAmpPercentagePD[CH14]", "0"], ["ElectrodeAmpPercentagePD[CH15]", "0"], ["ElectrodeAmpPercentagePD[CH16]", "0"], ["ElectrodeAmpPercentagePD[CH17]", "0"], ["ElectrodeAmpPercentagePD[CH18]", "0"], ["ElectrodeAmpPercentagePD[CH19]", "0"], ["ElectrodeAmpPercentagePD[CH20]", "0"], ["ElectrodeAmpPercentagePD[CH21]", "0"], ["ElectrodeAmpPercentagePD[CH22]", "0"], ["ElectrodeAmpPercentagePD[CH23]", "0"], ["ElectrodeAmpPercentagePD[CH24]", "0"], ["ElectrodeAmpPercentagePD[CH25]", "0"], ["ElectrodeAmpPercentagePD[CH26]", "0"]]
  # "PATIENT STIM STRUCTURE"
  # "SWEX 0091  Rev 1.8"
  # "Instructions\n1) Copy clipboard from Excel to Import Control.\n2) Run VI.\n3) Edit - Make Current Values Defaults.\n4) Save VI.\n5) Copy tables to new VIs."
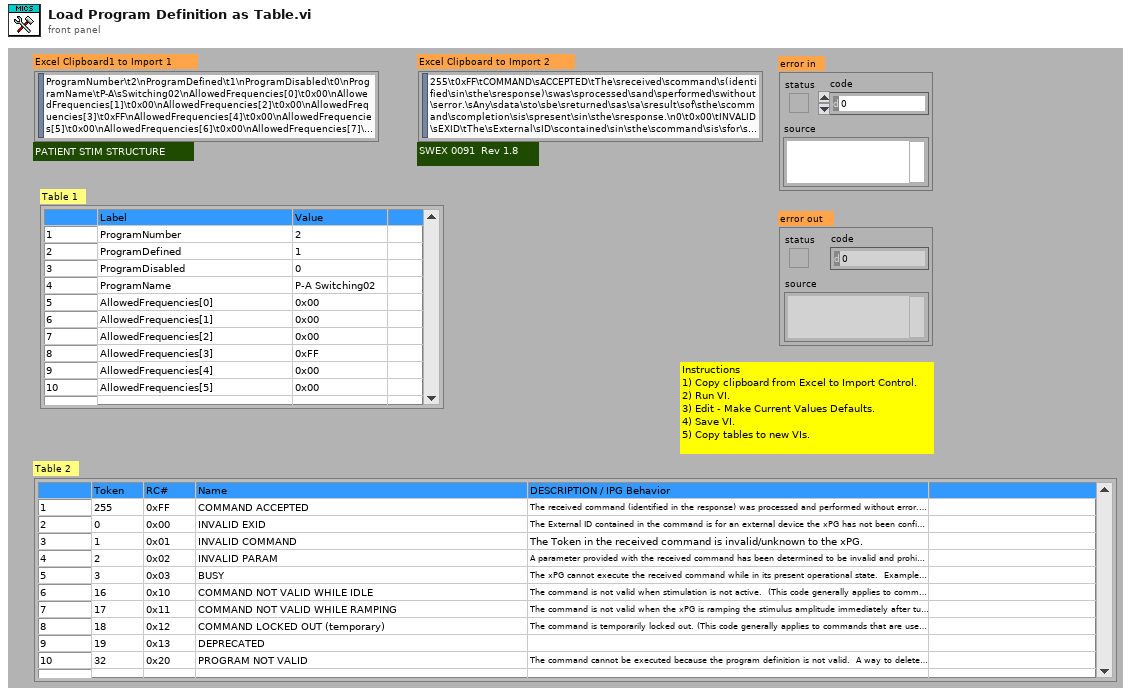
[diagram p1: front panel]
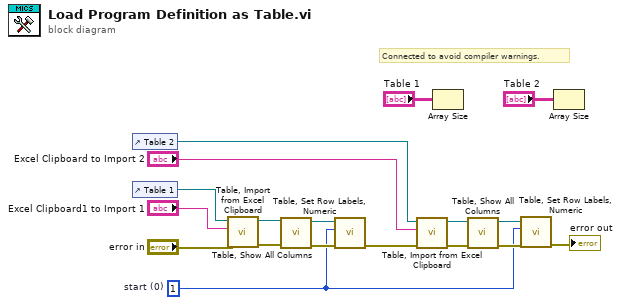
[diagram p0: block diagram]
diagram:
  w3 = 1  # start (0)
  # "Connected to avoid compiler warnings."
  n1 = control-ref of="Table 2"() -> (w5:refnum<vi>)
  n2 = control-ref of="Table 1"() -> (w17:refnum<vi>)
  n3 = call "Table, Import from Excel Clipboard.vi"("error in"="error in", "Excel Clipboard to Import"="Excel Clipboard1 to Import 1", "Tbl Refnum"=w17) -> ("error out"=w15:errorcluster, "Tbl Refnumout"=w16:refnum<vi>)  [unwired: 7 in]
  n4 = call "Table, Show All Columns.vi"("error in"=w15, "Tbl Refnum"=w16) -> ("error out"=w13:errorcluster, "Tbl Refnum out"=w12:refnum<vi>)  [unwired: 8 in]
  n5 = call "Table, Set Row Labels, Numeric.vi"("error in"=w13, "start (0)"=w3, "Tbl Refnum"=w12) -> ("error out"=w11:errorcluster)  [unwired: 7 in, 1 out]
  n6 = call "Table, Import from Excel Clipboard.vi"("error in"=w11, "Excel Clipboard to Import"="Excel Clipboard to Import 2", "Tbl Refnum"=w5) -> ("error out"=w10:errorcluster, "Tbl Refnumout"=w2:refnum<vi>)  [unwired: 7 in]
  n7 = Array Size(array="Table 1") -> ()  [unwired: 1 out]
  n8 = call "Table, Show All Columns.vi"("error in"=w10, "Tbl Refnum"=w2) -> ("error out"=w9:errorcluster, "Tbl Refnum out"=w1:refnum<vi>)  [unwired: 8 in]
  n9 = call "Table, Set Row Labels, Numeric.vi"("error in"=w9, "start (0)"=w3, "Tbl Refnum"=w1) -> ("error out"=→"error out":errorcluster)  [unwired: 7 in, 1 out]
  n10 = Array Size(array="Table 2") -> ()  [unwired: 1 out]
